vi "Translate to Array Data_BU4.vi"(0 "original data":path=path "C:/Users/User/Desktop/aaa.csv", 1 "Only Use Last Value?":bool=TRUE, 2 "Electrode number, N":u16=8, 3 "Current Mode":u8[][](array[numeric]), 5 "original error":errorcluster, 7 "Array Mode":u16(ring) items=["None", "Gradient + Dipole dipole", "Gradient", "Dipole Dipole", "Schlumberger"], 9 "modified data":path=path "C:/Users/User/Desktop/test.csv", 11 "modified error":errorcluster, 12 "Inverse\nPolarity":bool=TRUE, 13 "Insert\nBreak":bool=TRUE) -> ()   [LabVIEW 2023]
uses:
  <vilib>/Utility/error.llb/DialogType.ctl
panel:
  in  "External\nRef":bool=TRUE
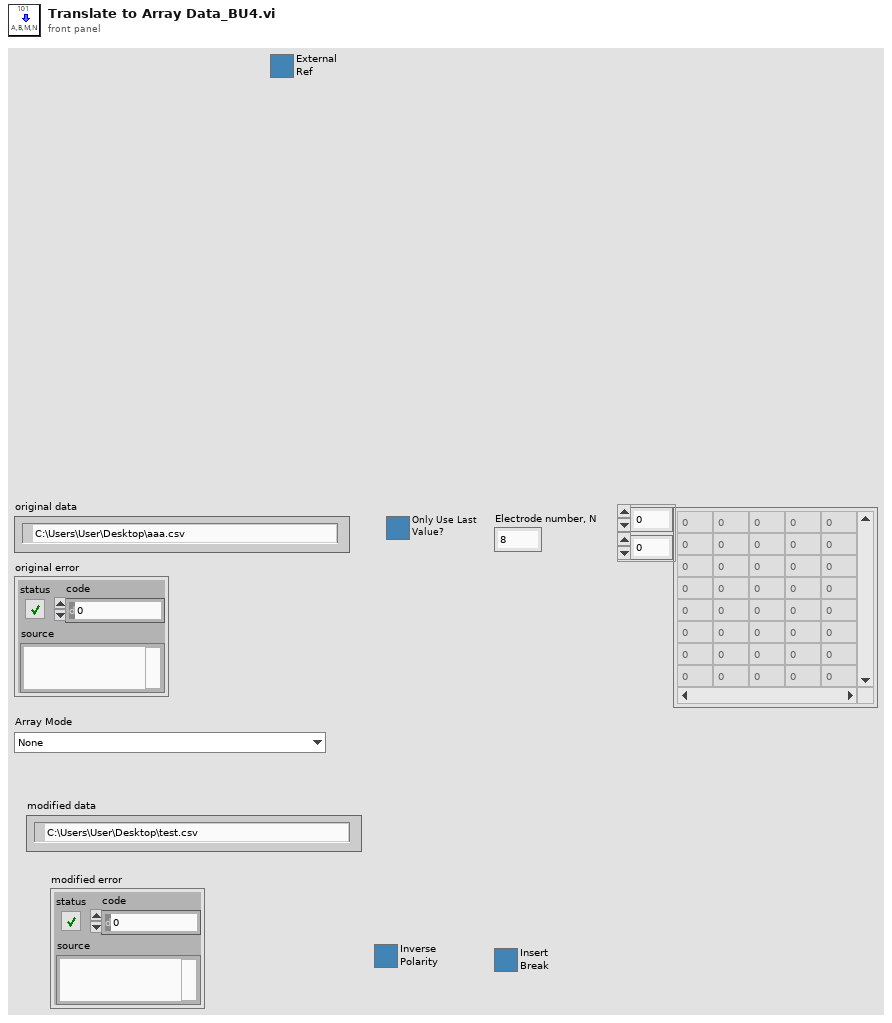
[diagram p1: front panel]
types:
  T1 = enum16{"open", "replace", "create", "open or create", "replace or create", "replace or create with confirmation"}
  T2 = typedef "DialogType.ctl" = u16
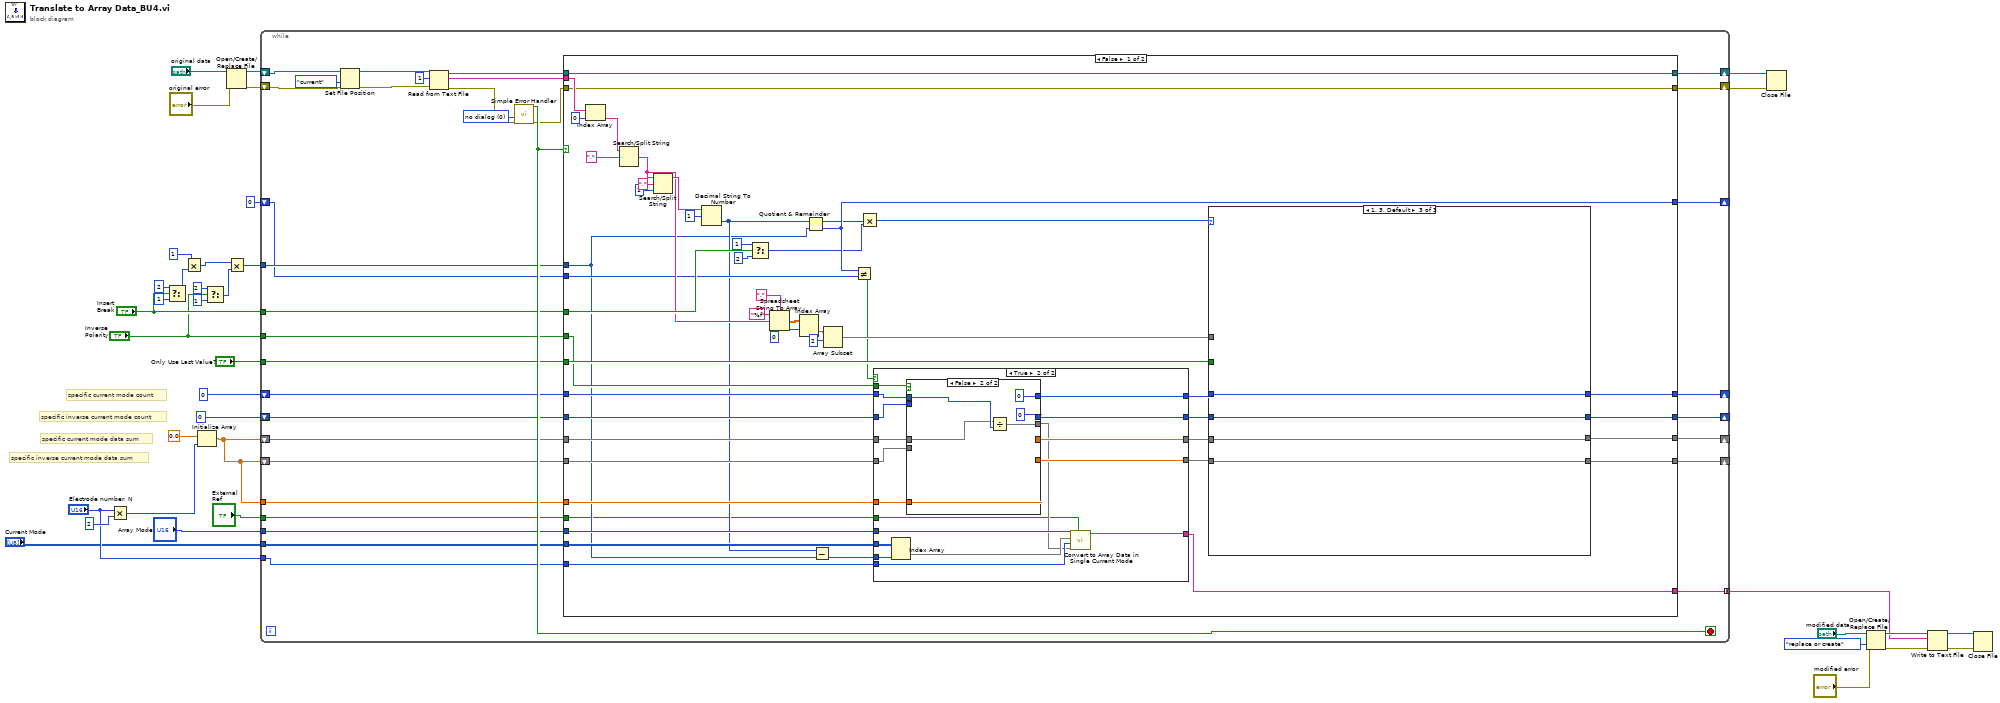
[diagram p0: block diagram]
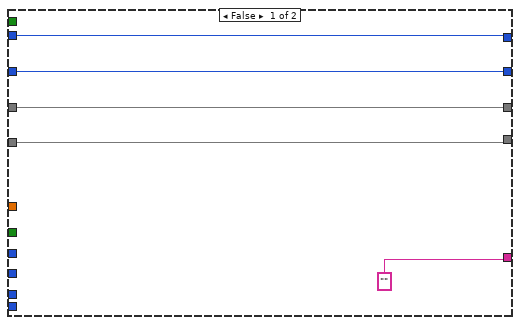
[diagram p2: hidden frame]
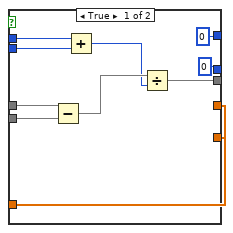
[diagram p3: hidden frame]
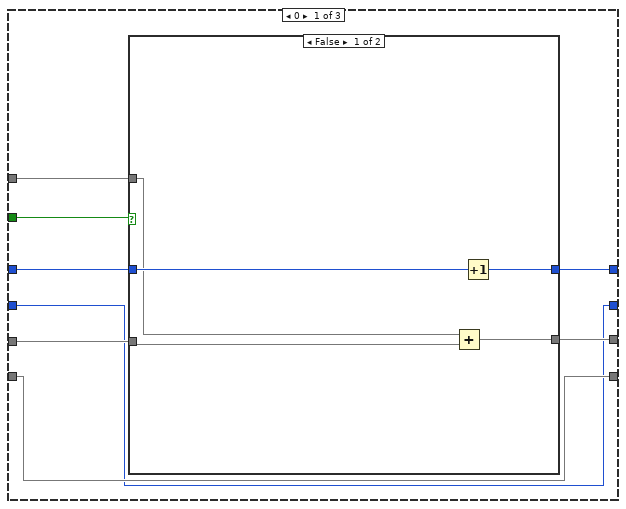
[diagram p4: hidden frame]
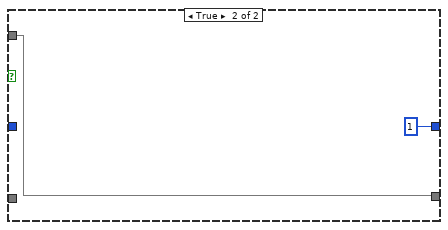
[diagram p5: hidden frame]
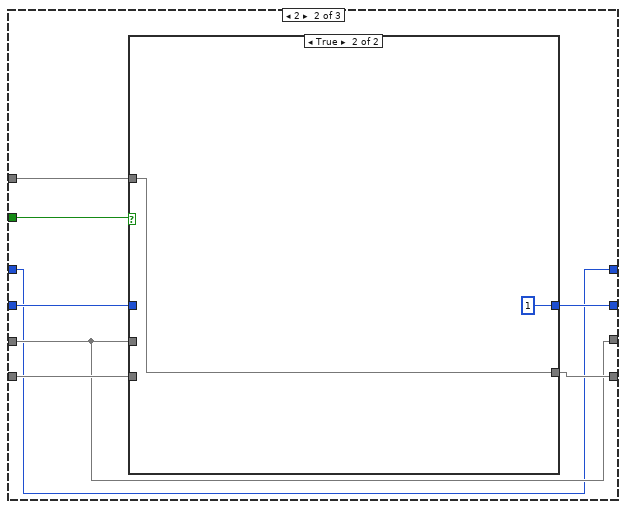
[diagram p6: hidden frame]
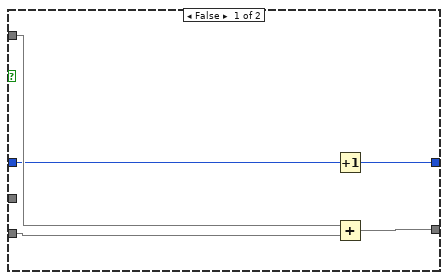
[diagram p7: hidden frame]
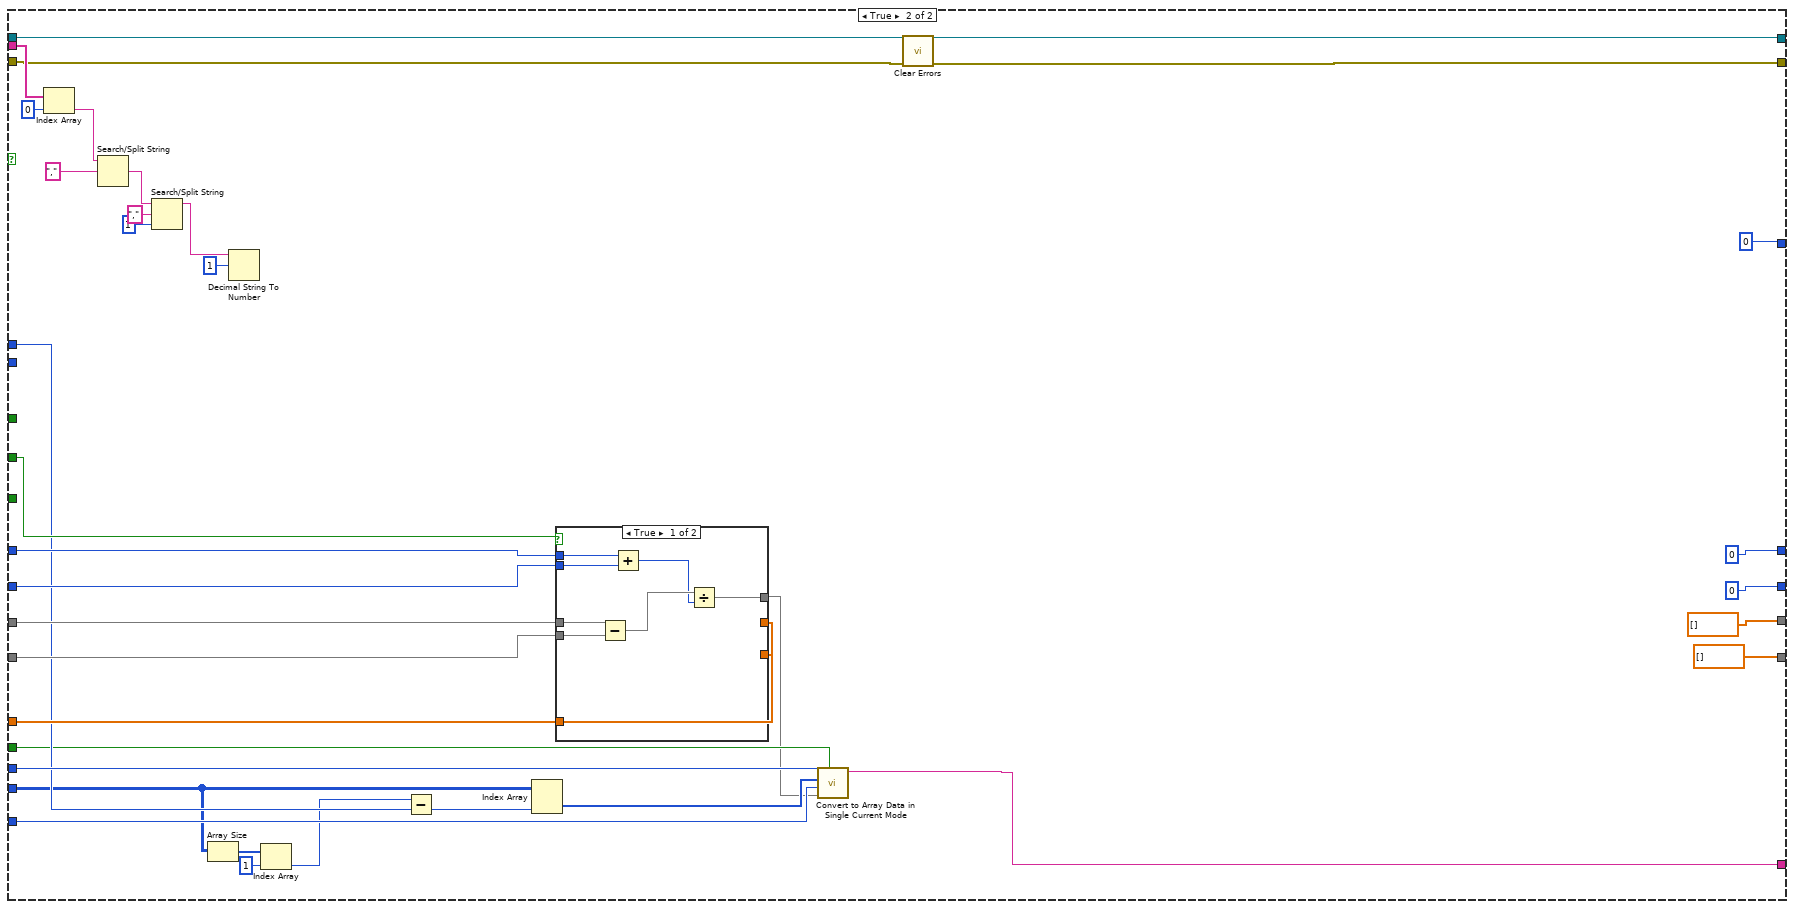
[diagram p8: hidden frame]
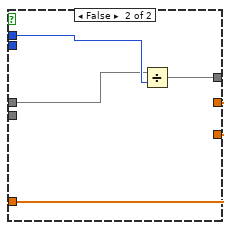
[diagram p9: hidden frame]
diagram:
  # "specific inverse current mode data sum"
  # "specific current mode data sum"
  # "specific inverse current mode count"
  # "specific current mode count"
  n1 = Multiply(x="Electrode number, N", y=u16 2) -> (x*y=w11:u16)
  n2 = Select(t=2 ("number"), s="Insert\nBreak", f=1 ("number")) -> (s? t:f=w20:i32)
  n3 = Multiply(x=1 ("number"), y=w20) -> (x*y=w14:i32)
  n4 = Initialize Array(0.0 ("element"), w11) -> (w10:dbl[])
  n5 = Select(t=2 ("number"), s="Inverse\nPolarity", f=1 ("number")) -> (s? t:f=w19:i32)
  n6 = Open/Create/Replace File(file path (use dialog)="original data", error in="original error") -> (refnum out=w34:refnum<file>, error out=w35:errorcluster)  [unwired: 4 in, 1 out]
  n7 = Multiply(x=w14, y=w19) -> (x*y=w18:i32)
  n8 = while {
    shift-right: [w63] -> w29
    shift-left: w35 -> [w70]
    shift-right: [w62] -> w36
    shift-left: w34 -> [w61]
    tunnel: "Insert\nBreak" -> [w57]
    tunnel: "Inverse\nPolarity" -> [w56]
    tunnel: "Only Use Last Value?" -> [w55]
    tunnel: w18 -> [w54]
    shift-right: [w49] -> _
    shift-left: 0 ("number") -> [w53]
    shift-right: [w46] -> _
    shift-left: 0 ("number") -> [w52]
    shift-right: [w48] -> _
    shift-left: w10 -> [w51]
    shift-right: [w47] -> _
    shift-left: w10 -> [w50]
    shift-right: [w45] -> _
    shift-left: 0 -> [w44]
    tunnel: w10 -> [w43]
    tunnel: "Current Mode" -> [w41]
    tunnel: "Array Mode" -> [w42]
    tunnel: "Electrode number, N" -> [w40]
    tunnel: "External\nRef" -> [w39]
    tunnel: [w38] -> w4 mode=concatenating
    stop <- w67 stop-if-true
    w68 = T2 0 items=["no dialog", "OK message", "continue or stop message", "OK message + warnings", "continue/stop + warnings"] ("type of dialog (OK msg:1)")
    n9 = Set File Position(refnum=w61, from (0:start)=enum16{"start", "end", "current"}."current", error in=w70) -> (refnum out=w60:refnum<file>, error out=w59:errorcluster)  [unwired: 1 in]
    n10 = Read from Text File(file (use dialog)=w60, count=1, error in=w59) -> (refnum out=w65:refnum<file>, text=w66:string[], error out=w64:errorcluster)  [unwired: 1 in, 1 out]
    n11 = call <vilib>:"Simple Error Handler.vi"("type of dialog (OK msg:1)"=w68, "error in (no error)"=w64) -> ("error?"=w67:bool, "error out"=w58:errorcluster)  [unwired: 3 in, 3 out]
    n12 = case shown="False" w67 {
      tunnel: w66 -> [w117 w225]
      tunnel: w65 -> [w114 w222]
      tunnel: w58 -> [w113 w202]
      tunnel: [w114 w222] -> w62
      tunnel: [w113 w201] -> w63
      tunnel: w57 -> [w110 _]
      tunnel: w56 -> [w89 w215]
      tunnel: w55 -> [w109 _]
      tunnel: w54 -> [w75 w211]
      tunnel: w53 -> [w93 w219]
      tunnel: w52 -> [w92 w218]
      tunnel: w51 -> [w91 w217]
      tunnel: w50 -> [w90 w216]
      tunnel: [w99 0 ("number")] -> w49
      tunnel: [w98 dbl[] [] ("subarray")] -> w48
      tunnel: [w97 dbl[] [] ("subarray")] -> w47
      tunnel: [w96 0 ("number")] -> w46
      tunnel: [w94 0] -> w45
      tunnel: w44 -> [w95 _]
      tunnel: w43 -> [w83 w214]
      tunnel: w42 -> [w79 w213]
      tunnel: w41 -> [w78 w198]
      tunnel: w40 -> [w74 w210]
      tunnel: w39 -> [w73 w209]
      tunnel: [w72 w208] -> w38
      frame False {
        n13 = Index Array(array=w117, index=0) -> (element=w115:string)
        n14 = Search/Split String(string=w115, search string/char (-)=",") -> (match + rest of string=w105:string)  [unwired: 1 in, 2 out]
        n15 = Search/Split String(string=w105, search string/char (-)=",", offset (0)=1) -> (substring before match=w106:string)  [unwired: 2 out]
        n16 = Decimal String To Number(string=w106, offset=1) -> (number=w76:i32)  [unwired: 1 in, 1 out]
        n17 = Select(t=1, s=w110, f=2 ("y")) -> (s? t:f=w82:i32)
        n18 = Spreadsheet String To Array(delimiter (Tab)=",", format string="%f", spreadsheet string=w105) -> (array=w104:dbl[][])  [unwired: 1 in]
        n19 = Index Array(array=w104, index (row)=0) -> (element=w102:dbl[])  [unwired: 1 in]
        n20 = Quotient & Remainder(x=w76, y=w75) -> (x-y*floor(x/y)=w81:i32, floor(x/y)=w94:i32)
        n21 = Subtract(x=w76, y=w75) -> (x-y=w77:i32)
        n22 = Array Subset(array=w102, index=2) -> (w100:dbl[])  [unwired: 1 in]
        n23 = Not Equal?(x=w94, y=w95) -> (x != y?=w84:bool)
        n24 = Multiply(x=w81, y=w82) -> (x*y=w80:i32)
        n25 = case shown="True" w84 {
          tunnel: w93 -> [w126 w141]
          tunnel: w92 -> [w125 w140]
          tunnel: w91 -> [w124 w143]
          tunnel: w90 -> [w123 w142]
          tunnel: w89 -> [_ w144]
          tunnel: [w126 w139] -> w88
          tunnel: [w125 w138] -> w87
          tunnel: [w124 w137] -> w86
          tunnel: [w123 w136] -> w85
          tunnel: w83 -> [_ w135]
          tunnel: w79 -> [_ w131]
          tunnel: w78 -> [_ w134]
          tunnel: w77 -> [_ w133]
          tunnel: w74 -> [_ w130]
          tunnel: w73 -> [_ w128]
          tunnel: ["" ("String") w127] -> w72
          frame False {
          }
          frame True {
            n26 = Index Array(array=w134, index (col)=w133) -> (element=w132:u8[])  [unwired: 1 in]
            n27 = case shown="False" w144 {
              tunnel: w143 -> [w154 w157]
              tunnel: w142 -> [w153 _]
              tunnel: w141 -> [w152 w158]
              tunnel: w140 -> [w151 _]
              tunnel: [0 ("number") 0 ("number")] -> w139
              tunnel: [0 ("number") 0 ("number")] -> w138
              tunnel: [w146 w156] -> w137
              tunnel: [w146 w156] -> w136
              tunnel: w135 -> [w146 w156]
              tunnel: [w145 w155] -> w129
              frame True {
                n28 = Subtract(x=w154, y=w153) -> (x-y=w150:dbl[])
                n29 = Add(x=w152, y=w151) -> (x+y=w149:i32)
                n30 = Divide(x=w150, y=w149) -> (x/y=w145:dbl[])
              }
              frame False {
                n31 = Divide(x=w157, y=w158) -> (x/y=w155:dbl[])
              }
            }
            n32 = call "Convert to Array Data in Single Current Mode.vi"("External\nRef"=w128, "data"=w129, "Electrode number, N"=w130, "Current Mode"=w132, "Array Mode"=w131) -> ("String"=w127:string)  [unwired: 6 in]
          }
        }
        n33 = case shown="1, 3, Default" w80 {
          tunnel: w109 -> [w168 w183 _]
          tunnel: w100 -> [w164 w182 _]
          tunnel: w88 -> [w167 w176 w194]
          tunnel: w87 -> [w161 w179 w193]
          tunnel: w86 -> [w166 w177 w192]
          tunnel: w85 -> [w162 w181 w191]
          tunnel: [w165 w176 w194] -> w99
          tunnel: [w163 w177 w192] -> w98
          tunnel: [w162 w180 w191] -> w97
          tunnel: [w161 w178 w193] -> w96
          frame 0 {
            n34 = case shown="False" w168 {
              tunnel: w167 -> [w173 _]
              tunnel: w166 -> [w170 _]
              tunnel: [w172 1 ("number")] -> w165
              tunnel: w164 -> [w169 w174]
              tunnel: [w171 w174] -> w163
              frame False {
                n35 = Add(x=w169, y=w170) -> (x+y=w171:dbl[])
                n36 = Increment(x=w173) -> (x+1=w172:i32)
              }
              frame True {
              }
            }
          }
          frame 2 {
            n37 = case shown="True" w183 {
              tunnel: w177 -> [_ _]
              tunnel: w182 -> [w187 w190]
              tunnel: [w188 w190] -> w180
              tunnel: w181 -> [w186 _]
              tunnel: w179 -> [w185 _]
              tunnel: [w184 1 ("number")] -> w178
              frame False {
                n38 = Increment(x=w185) -> (x+1=w184:i32)
                n39 = Add(x=w187, y=w186) -> (x+y=w188:dbl[])
              }
              frame True {
              }
            }
          }
          frame 1, 3, Default {
          }
        }
      }
      frame True {
        n40 = Index Array(array=w225, index=0) -> (element=w223:string)
        n41 = Search/Split String(string=w223, search string/char (-)=",") -> (match + rest of string=w220:string)  [unwired: 1 in, 2 out]
        n42 = Search/Split String(string=w220, search string/char (-)=",", offset (0)=1) -> (substring before match=w221:string)  [unwired: 2 out]
        n43 = Array Size(array=w198) -> (size(s)=w197:i32[])
        n44 = Decimal String To Number(string=w221, offset=1) -> ()  [unwired: 1 in, 2 out]
        n45 = Index Array(array=w197, index=1) -> (element=w195:i32)
        n46 = Subtract(x=w195, y=w211) -> (x-y=w212:i32)
        n47 = Index Array(array=w198, index (col)=w212) -> (element=w200:u8[])  [unwired: 1 in]
        n48 = case shown="True" w215 {
          tunnel: w217 -> [w237 w240]
          tunnel: w216 -> [w236 _]
          tunnel: w219 -> [w235 w241]
          tunnel: w218 -> [w234 _]
          tunnel: [w231 w239] -> _
          tunnel: [w231 w239] -> _
          tunnel: w214 -> [w231 w239]
          tunnel: [w230 w238] -> w199
          frame True {
            n49 = Subtract(x=w237, y=w236) -> (x-y=w233:dbl[])
            n50 = Add(x=w235, y=w234) -> (x+y=w232:i32)
            n51 = Divide(x=w233, y=w232) -> (x/y=w230:dbl[])
          }
          frame False {
            n52 = Divide(x=w240, y=w241) -> (x/y=w238:dbl[])
          }
        }
        n53 = call "Convert to Array Data in Single Current Mode.vi"("External\nRef"=w209, "data"=w199, "Electrode number, N"=w210, "Current Mode"=w200, "Array Mode"=w213) -> ("String"=w208:string)  [unwired: 6 in]
        n54 = call <vilib>:"Clear Errors.vi"("error in (no error)"=w202) -> ("error out"=w201:errorcluster)  [unwired: 5 in, 1 out]
      }
    }
  }
  n55 = Close File(refnum=w36, error in=w29) -> ()  [unwired: 2 out]
  n56 = Open/Create/Replace File(file path (use dialog)="modified data", error in="modified error", operation (0:open)=T1."replace or create") -> (refnum out=w6:refnum<file>, error out=w5:errorcluster)  [unwired: 3 in, 1 out]
  n57 = Write to Text File(file (use dialog)=w6, text=w4, error in=w5) -> (refnum out=w3:refnum<file>, error out=w2:errorcluster)  [unwired: 1 in, 1 out]
  n58 = Close File(refnum=w3, error in=w2) -> ()  [unwired: 2 out]
